vi "CheckDataQueue.vi"(8 "error in (no error)":errorcluster, 11 "data Q":refnum<queue>) -> (0 "error out":errorcluster, 2 "ready":bool, 3 "data":variant)   [LabVIEW 2017, in "FileManager.lvlib"]
uses:
  <vilib>/addons/InsightCM/Devices/Shared/Common/FileManager/FileManager.lvlib
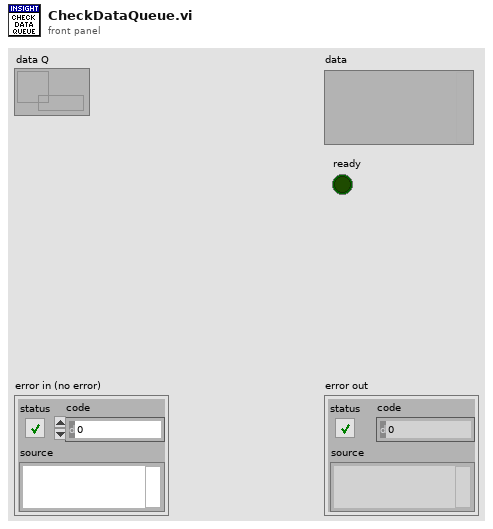
[diagram p1: front panel]
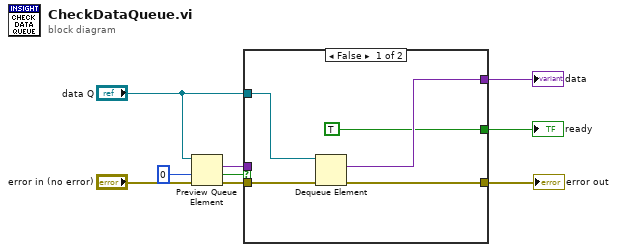
[diagram p0: block diagram]
diagram:
  n1 = Preview Queue Element(queue="data Q", timeout in ms (-1)=0, error in (no error)="error in (no error)") -> (element=w6:variant, timed out?=w7:bool, error out=w5:errorcluster)  [unwired: 1 out]
  n2 = case shown="False" w7 {
    tunnel: w6 -> [_ _]
    tunnel: w5 -> [w14 w15]
    tunnel: "data Q" -> [w13 _]
    tunnel: [w12 _] -> w2
    tunnel: [TRUE _] -> w3
    tunnel: [w10 w15] -> w1
    frame False {
      n3 = Dequeue Element(queue=w13, error in (no error)=w14) -> (element=w12:variant, error out=w10:errorcluster)  [unwired: 1 in, 2 out]
    }
    frame True {
    }
  }
  "error out" <- w1
  "data" <- w2
  "ready" <- w3
